vi "Stop Core.vi"(10 "final error code":i32, 11 "Display Console in":refnum<class "Sensor Interface.lvclass">) -> (3 "Display Console out":refnum<class "Sensor Interface.lvclass">)   [LabVIEW 2019, in "Sensor Interface Actor.lvlib" / "Sensor Interface.lvclass"]
doc: "(<B>Filename</B>: Actor Framework.lvlib:Actor.lvclass:Stop Core.vi)\n\nDefines what the actor does before it stops. Use the <B>final error code</B> input to determine whether the actor shut down in response to an error.\n\nBy default, this method passes the Stop message along to all auto-stop nested actors. A descendant class may override this method to define additional behavior, such as shutting down any processes the actor initiated in its override of the Actor Core method."
uses:
  Sensor Interface.lvclass
  Sensor Interface.lvclass/Sensor Interface.ctl
  Abstract Sensor Interface Actor/Abstract Sensor Interface/Abstract Sensor Interface.lvclass
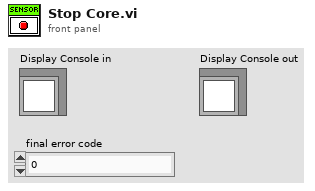
[diagram p1: front panel]
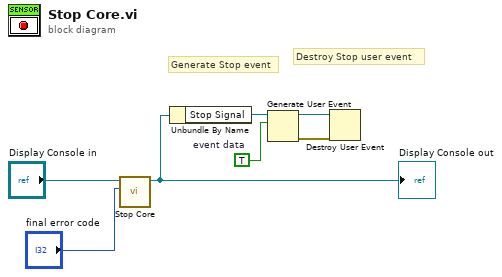
[diagram p0: block diagram]
diagram:
  w1 = TRUE  # event data
  # "Destroy Stop user event"
  # "Generate Stop event"
  n1 = call-parent "Stop Core.vi"("final error code"="final error code", "Actor in"="Display Console in") -> ("Actor out"=w2:refnum<class "Sensor Interface.lvclass">)  [unwired: 9 in]
  "Display Console out" <- w2
  n2 = Unbundle By Name(w2) -> ("Stop Signal"=w5:refnum<user-event>)
  n3 = Generate User Event(user event=w5, event data cluster=w1) -> (user event out=w3:refnum<user-event>, error out=w4:errorcluster)  [unwired: 2 in]
  n4 = Destroy User Event(user event=w3, error in=w4) -> ()  [unwired: 1 out]
